vi "roboRIO v1.0 Read Accelerometer.vi"(8 "error in (no error)":errorcluster, 9 "LSB Weight (g-force/bit)":dbl, 10 "Channel List":T3, 11 "myRIO Ref In":T1) -> (0 "error out":errorcluster, 2 "dbl Scaled Value List":dbl[](array[numeric]), 3 "myRIO Ref Out":T1)   [LabVIEW 2021]
uses:
  <vilib>/myRIO/Common/Instrument Driver Framework/myRIO v1.0/Accelerometer/typedefs/Accelerometer Channels List.ctl
  <vilib>/myRIO/Common/Instrument Driver Framework/myRIO v1.0/Accelerometer/typedefs/Accelerometer Channels Enum.ctl
  <vilib>/myRIO/Common/Instrument Driver Framework/Utilities/typedefs/myRIO v1.0 Reference.ctl
  <vilib>/myRIO/Common/Instrument Driver Framework/Utilities/typedefs/Generic FPGA Reference.ctl
  <vilib>/myRIO/Common/Instrument Driver Framework/roboRIO v1.0/Accelerometer/typedefs/roboRIO Accelerometer FPGA Reference.ctl
  <vilib>/rvi/errors/niLvFpgaAdjustHostInterfaceError.vi
  <vilib>/rvi/interface/nirviReadWriteControl/nirviReadWriteControl.xnode
  <vilib>/rvi/interface/Simulation/niFpgaSimulationCallBeginRW.vi
  NiFpgaLv.dll
panel:
  # "This VI reads one analog value from a user specified analog channel on\nthe myRIO v1.0 hardware. The value is read on the FPGA as a u16 and \nscaled to a dbl based on the specifications of the ADC. Please see Block Diagram for details."
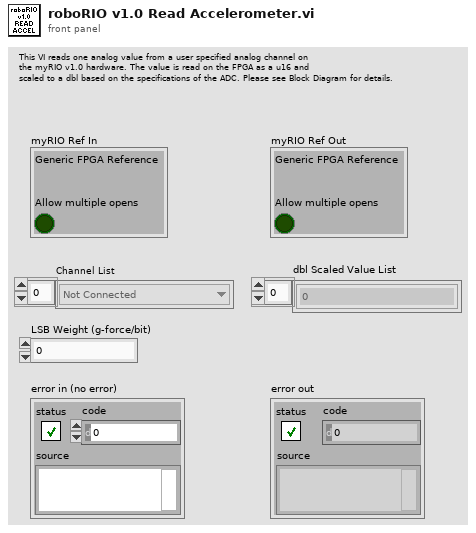
[diagram p1: front panel]
types:
  T1 = typedef "myRIO v1.0 Reference.ctl" = cluster{"Generic FPGA Reference":T2, "Allow multiple opens":bool}
  T2 = typedef "Generic FPGA Reference.ctl" = refnum<k20>
  T3 = typedef "Accelerometer Channels List.ctl" = T4[]
  T4 = typedef "Accelerometer Channels Enum.ctl" = enum16{"Not Connected", "X-Axis", "Y-Axis", "Z-Axis"}
  T5 = typedef "roboRIO Accelerometer FPGA Reference.ctl" = refnum<k20>
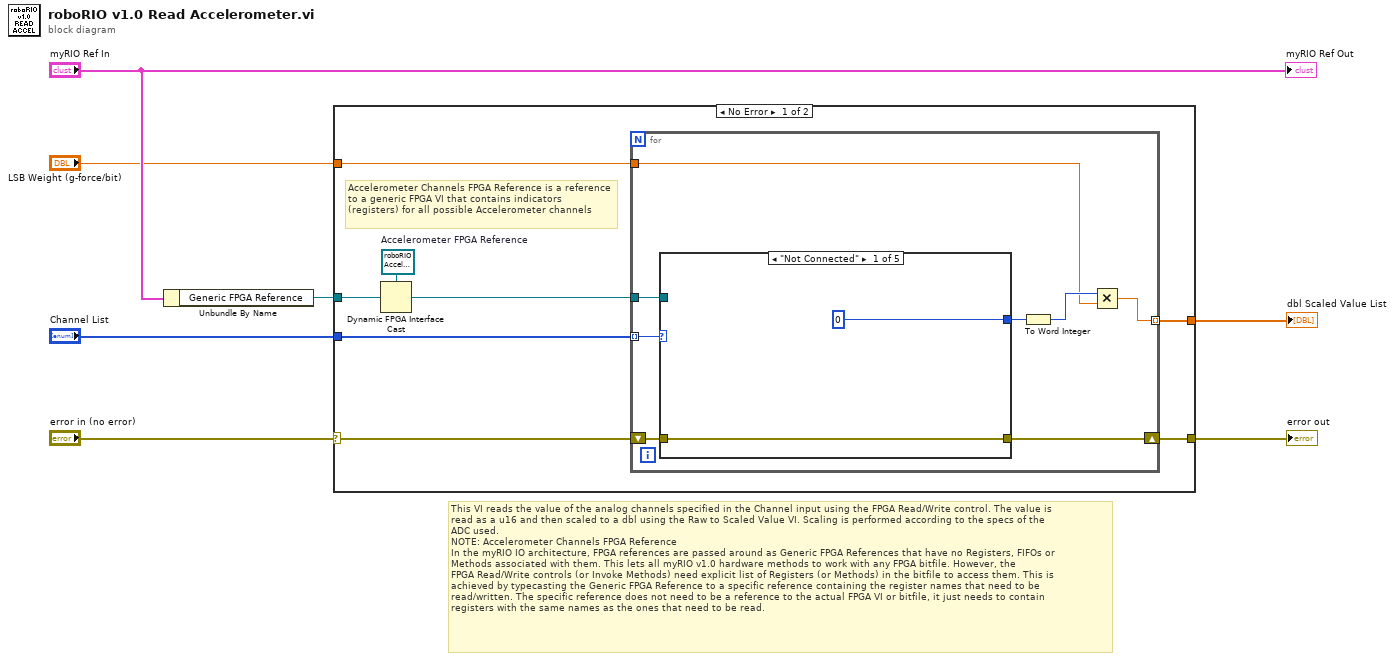
[diagram p0: block diagram]
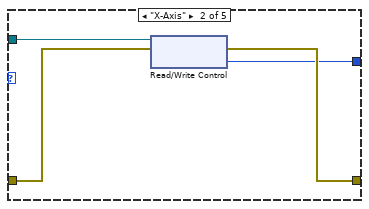
[diagram p2: hidden frame]
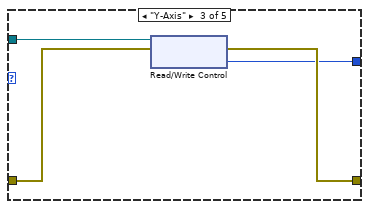
[diagram p3: hidden frame]
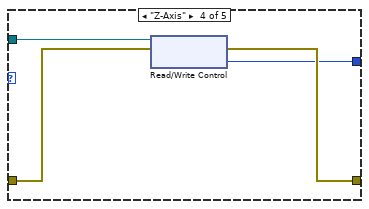
[diagram p4: hidden frame]
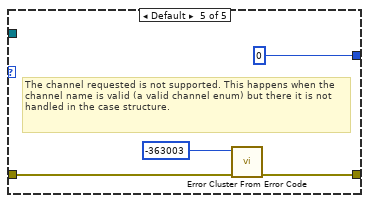
[diagram p5: hidden frame]
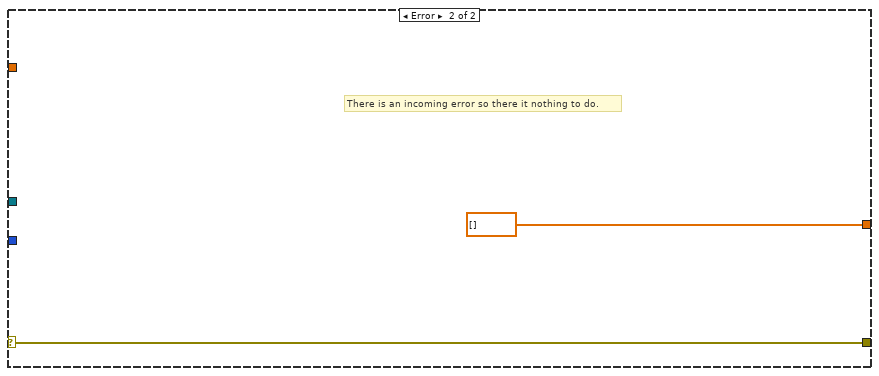
[diagram p6: hidden frame]
diagram:
  # "This VI reads the value of the analog channels specified in the Channel input using the FPGA Read/Write control. The value is \nread as a u16 and then scaled to a dbl using the Raw to Scaled Value VI. Scaling is performed according to the specs of the \nADC used.\nNOTE: Accelerometer Channels FPGA Reference\nIn the myRIO IO architecture, FPGA references are passed around as Generic FPGA References that have no Registers, FIFOs or\nMethods associated with them. This lets all myRIO v1.0 hardware methods to work with any FPGA bitfile. However, the \nFPGA Read/Write controls (or Invoke Methods) need explicit list of Registers (or Methods) in the bitfile to access them. This is \nachieved by typecasting the Generic FPGA Reference to a specific reference containing the register names that need to be \nread/written. The specific reference does not need to be a reference to the actual FPGA VI or bitfile, it just needs to contain \nregisters with the same names as the ones that need to be read."
  n1 = Unbundle By Name("myRIO Ref In") -> ("Generic FPGA Reference"=w2:T2)
  n2 = case shown="No Error" "error in (no error)" {
    selector: "error in (no error)" -> [w9 w43]
    tunnel: w2 -> [w13 _]
    tunnel: [w12 w43] -> w7
    tunnel: [w11 dbl[] []] -> w6
    tunnel: "Channel List" -> [w10 _]
    tunnel: "LSB Weight (g-force/bit)" -> [w8 _]
    frame No Error {
      w15 = T5 refnum  # Accelerometer FPGA Reference
      # "Accelerometer Channels FPGA Reference is a reference to a generic FPGA VI that contains indicators (registers) for all possible Accelerometer channels"
      n3 = Dynamic FPGA Interface Cast(Session In=w15, Type=w13) -> (Session Out=w14:T5)
      n4 = for {
        tunnel: w14 -> [w23]
        shift-right: [w21] -> w12
        shift-left: w9 -> [w22]
        tunnel: w10 -> [w20] mode=indexing
        tunnel: [w17] -> w11 mode=indexing
        tunnel: w8 -> [w16]
        n5 = case shown="\"Not Connected\"" w20 {
          tunnel: w22 -> [w25 w29 w33 w37 w38]
          tunnel: [w25 w28 w32 w36 w39] -> w21
          tunnel: [u16 0 ("AI7") w27 w31 w35 u16 0 ("AI7")] -> w19
          tunnel: w23 -> [_ w26 w30 w34 _]
          frame "Not Connected" {
          }
          frame "X-Axis" {
            n6 = xnode "Read/Write Control"("FPGA VI Reference In"=w26, "error in"=w29) -> ("error out"=w28:errorcluster, "ACC.X.VAL"=w27:u16)  [unwired: 1 out]
          }
          frame "Y-Axis" {
            n7 = xnode "Read/Write Control"("FPGA VI Reference In"=w30, "error in"=w33) -> ("error out"=w32:errorcluster, "ACC.Y.VAL"=w31:u16)  [unwired: 1 out]
          }
          frame "Z-Axis" {
            n8 = xnode "Read/Write Control"("FPGA VI Reference In"=w34, "error in"=w37) -> ("error out"=w36:errorcluster, "ACC.Z.VAL"=w35:u16)  [unwired: 1 out]
          }
          frame Default {
            # "The channel requested is not supported. This happens when the channel name is valid (a valid channel enum) but there it is not handled in the case structure."
            n9 = call <vilib>:"Error Cluster From Error Code.vi"("error in (no error)"=w38, "error code (0)"=-363003) -> ("error out"=w39:errorcluster)  [unwired: 7 in]
          }
        }
        n10 = To Word Integer(number=w19) -> (16bit integer=w18:i16)
        n11 = Multiply(x=w18, y=w16) -> (x*y=w17:dbl)
      }
    }
    frame Error {
      # "There is an incoming error so there it nothing to do."
    }
  }
  "error out" <- w7
  "dbl Scaled Value List" <- w6
  "myRIO Ref Out" <- "myRIO Ref In"
